vi "计算距离.vi"(8 "error in (no error)":errorcluster caption="错误输入（无错误）", 11 "Navigation 输入":refnum<class "Navigation.lvclass">) -> (0 "error out":errorcluster caption="错误输出", 3 "Navigation 输出":refnum<class "Navigation.lvclass">)   [LabVIEW 2018, in "Navigation.lvclass"]
uses:
  Navigation.lvclass
  Navigation.lvclass/Navigation.ctl
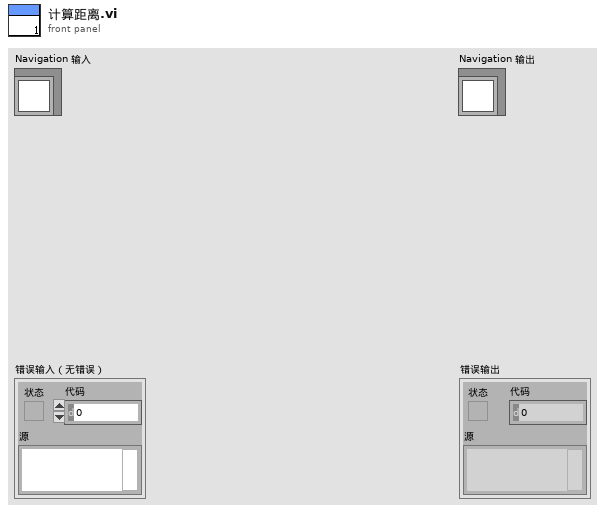
[diagram p1: front panel]
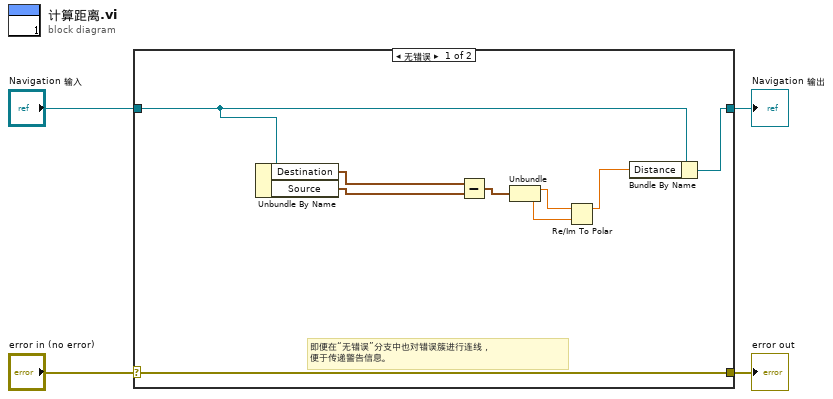
[diagram p0: block diagram]
diagram:
  n1 = case shown="无错误" "error in (no error)" {
    selector: "error in (no error)" -> [w13 w15]
    tunnel: [w13 w15] -> w3
    tunnel: [w5 w14] -> w1
    tunnel: "Navigation 输入" -> [w7 w14]
    frame No Error {
      # "即便在“无错误”分支中也对错误簇进行连线，\n便于传递警告信息。"
      n2 = Unbundle By Name(w7) -> ("Destination"=w12:cluster{"X":dbl, "Y":dbl}, "Source"=w11:cluster{"X":dbl, "Y":dbl})
      n3 = Subtract(x=w12, y=w11) -> (x-y=w10:cluster{"X":dbl, "Y":dbl})
      n4 = Unbundle(w10) -> ("X"=w9:dbl, "Y"=w8:dbl)
      n5 = Re/Im To Polar(2:w8, 3:w9) -> (1:w6:dbl)  [unwired: 1 out]
      n6 = Bundle By Name(cluster=w7, "Distance"=w6) -> (w5:refnum<class "Navigation.lvclass">)
    }
    frame Error {
    }
  }
  "error out" <- w3
  "Navigation 输出" <- w1
